vi "Add Label Parameters as Channels.vi"(6 "channel type":T1, 7 "highlight (F)":bool, 8 "error in":errorcluster, 9 "label parameters":T3, 10 "label name":string, 11 "frame ref":T2 format="%.0x") -> (0 "error out":errorcluster, 3 "channel refs":T2[](array[typedef]) format="%.0x")   [LabVIEW 2020, in "Communication Bus Template Scripting.lvlib"]
uses:
  Communication Bus Template Scripting.lvlib
  <vilib>/NI VeriStand/Custom Device API/Custom Device Item Ref.ctl
  Shared/VS Channels Definition for Label.ctl
  Shared/VS Channel Definition for Parameter.ctl
  Shared/Parameter Definition.ctl
  Encoding and Decoding/Encoding.ctl
  <vilib>/NI VeriStand/Custom Device API/Custom Device Channel Type.ctl
  Constants.vi
  <vilib>/NI VeriStand/Custom Device API/Custom Device API.lvlib
  Encoding and Decoding/Encoding and Decoding.lvlib
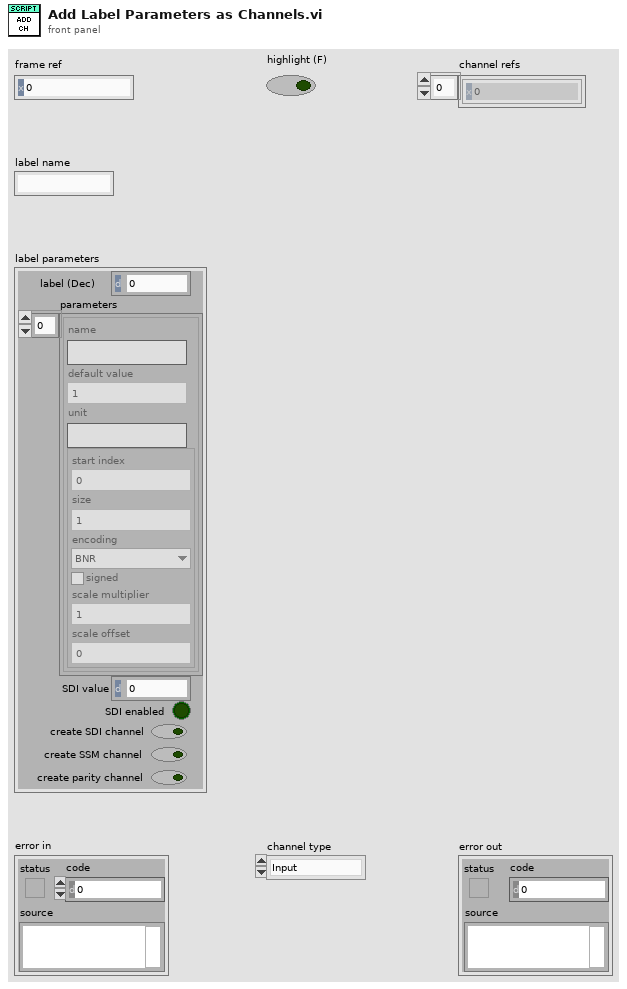
[diagram p1: front panel]
types:
  T1 = typedef "Custom Device API.lvlib/Custom Device Channel Type.ctl" = enum16{"Input", "Output"}
  T2 = typedef "Custom Device API.lvlib/Custom Device Item Ref.ctl" = u64
  T3 = typedef "VS Channels Definition for Label.ctl" = cluster{"label (Dec)":i32, "parameters":T4[], "SDI value":u8, "SDI enabled":bool, "create SDI channel":bool, "create SSM channel":bool, "create parity channel":bool}
  T4 = typedef "VS Channel Definition for Parameter.ctl" = cluster{"name":string, "default value":dbl, "unit":string, "Parameter":T5}
  T5 = typedef "Parameter Definition.ctl" = cluster{"start index":i32, "size":i32, "encoding":T6, "signed":bool, "scale multiplier":dbl, "scale offset":dbl}
  T6 = typedef "Encoding and Decoding.lvlib/Encoding.ctl" = enum16{"BNR", "BCD", "Discrete"}
  T7 = typedef "Custom Device API.lvlib/Custom Device Channel.ctl" = cluster{"Type":T1, "Units":string, "Default Value":dbl, "Faultable":bool, "Scalable":bool}
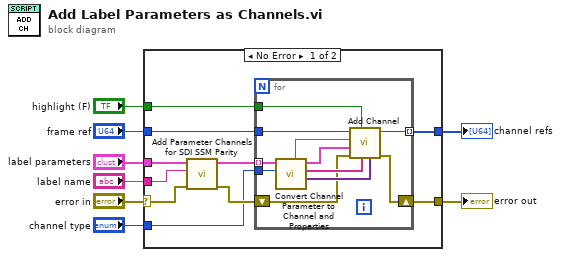
[diagram p0: block diagram]
diagram:
  n1 = case shown="No Error" "error in" {
    selector: "error in" -> [w12 w30]
    tunnel: [w18 w30] -> w7
    tunnel: "frame ref" -> [w17 _]
    tunnel: [w16 _] -> w2
    tunnel: "label parameters" -> [w14 _]
    tunnel: "highlight (F)" -> [w15 _]
    tunnel: "label name" -> [w10 _]
    tunnel: "channel type" -> [w9 _]
    frame No Error {
      n2 = call "Add Parameter Channels for SDI SSM Parity.vi"("error in"=w12, "label name"=w10, "label parameters"=w14) -> ("error out"=w11:errorcluster, "parameters in word"=w13:T4[])  [unwired: 7 in]
      n3 = for {
        tunnel: w15 -> [w21]
        shift-right: [w27] -> w18
        shift-left: w11 -> [w20]
        tunnel: w17 -> [w28]
        tunnel: [w26] -> w16 mode=indexing
        tunnel: w13 -> [w29] mode=indexing
        tunnel: w9 -> [w19]
        n4 = call "Convert Channel Parameter to Channel and Properties.vi"("channel type"=w19, "channel parameter"=w29) -> ("property values"=w22:variant[], "property names"=w23:string[], "channel"=w24:T7, "name"=w25:string)  [unwired: 6 in]
        n5 = call "Add Channel.vi"("Property Values"=w22, "Property names"=w23, "Highlight? (F)"=w21, "error in"=w20, "Channel"=w24, "Name"=w25, "Frame Ref"=w28) -> ("error out"=w27:errorcluster, "Channel Ref out"=w26:T2)  [unwired: 3 in]
      }
    }
    frame Error {
    }
  }
  "error out" <- w7
  "channel refs" <- w2
